vi "Find Attribute Match.vi"(10 "Attributes":refnum<class "Attribute.lvclass">[](array[class]), 11 "Attribute in":refnum<class "Attribute.lvclass">) -> (1 "Matched index":i32, 2 "Attributes dup":refnum<class "Attribute.lvclass">[](array[class]), 3 "Attribute out":refnum<class "Attribute.lvclass">)   [LabVIEW 2013, in "Attribute.lvclass"]
uses:
  Attribute.lvclass
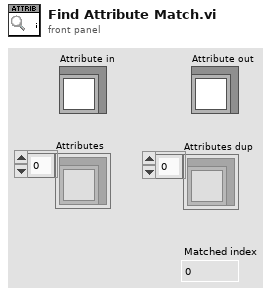
[diagram p1: front panel]
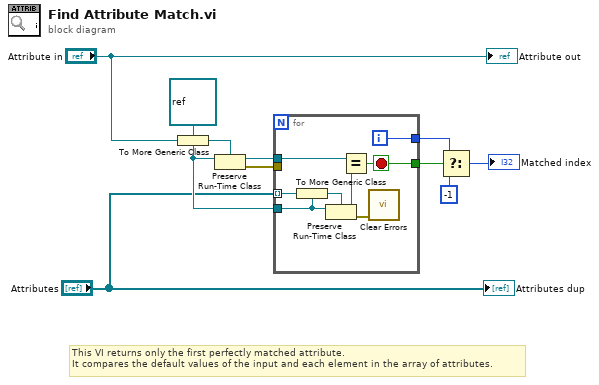
[diagram p0: block diagram]
diagram:
  w10 = refnum<class> refnum ("LabVIEW Object")
  # "This VI returns only the first perfectly matched attribute.\nIt compares the default values of the input and each element in the array of attributes."
  n1 = To More Generic Class(target class=w10, reference="Attribute in") -> (generic class reference=w5:refnum<class>)
  n2 = Preserve Run-Time Class(object in=w10, 2:w5) -> (object out=w3:refnum<class>, error out=w4:errorcluster)  [unwired: 1 in]
  n3 = for {
    tunnel: "Attributes" -> [w18] mode=indexing
    tunnel: w3 -> [w16]
    tunnel: w4 -> [_]
    tunnel: [w14] -> w6
    tunnel: [w13] -> w8
    tunnel: w10 -> [w12]
    i -> [w13]
    stop <- w14 stop-if-true
    n4 = To More Generic Class(target class=w12, reference=w18) -> (generic class reference=w17:refnum<class>)
    n5 = Preserve Run-Time Class(object in=w12, 2:w17) -> (object out=w15:refnum<class>, error out=w11:errorcluster)  [unwired: 1 in]
    n6 = Equal?(x=w16, y=w15) -> (x = y?=w14:bool)
    n7 = call <vilib>:"Clear Errors.vi"("error in (no error)"=w11) -> ()  [unwired: 6 in, 1 out]
  }
  n8 = Select(t=w8, s=w6, f=-1 ("t")) -> (s? t:f=→"Matched index":i32)
  "Attributes dup" <- "Attributes"
  "Attribute out" <- "Attribute in"
